vi "ECU Events Page.vi"(8 "error in (no error)":errorcluster, 11 "Node Ptr":T1 format="%.0x") -> (0 "error out":errorcluster)   [LabVIEW 2011, in "Engine Sim System Explorer.lvlib"]
uses:
  Engine Sim System Explorer.lvlib
  <vilib>/NI Veristand/Custom Device API/Custom Device Item Ref.ctl
  Shared/Engine Simulation Global.vi
  <vilib>/NI Veristand/Custom Device API/Get Item Property (Double).vi
  <vilib>/NI Veristand/Custom Device API/Set Item Property (Double).vi
  <vilib>/NI Veristand/Custom Device API/Custom Device API.lvlib
  Engine Simulation Shared.lvlib
panel:
  in  "FPGA Event Loop Rate (Hz)":dbl format="%#_p"
  in  "SHDocVw.IWebBrowser2":refnum<k7>(container)
  # "(Can be overriden per event on that event's page)"
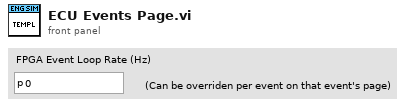
[diagram p1: front panel]
types:
  T1 = typedef "Custom Device API.lvlib/Custom Device Item Ref.ctl" = u64
  T2 = typedef "Custom Device API.lvlib/Custom Device Commands.ctl" = enum16{"Default", "Item renamed", "Shutdown", "Dynamic button pressed"}
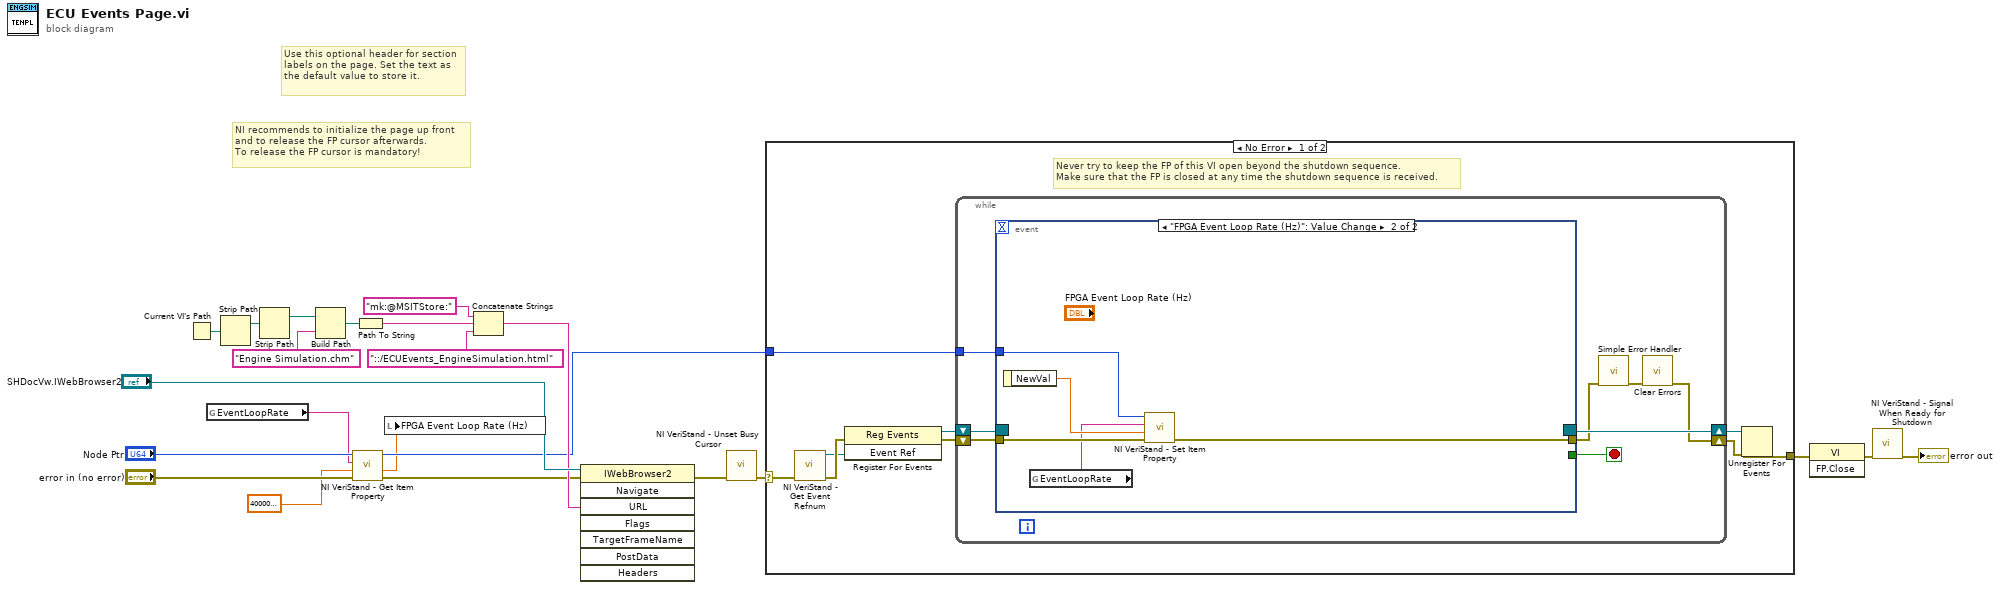
[diagram p0: block diagram]
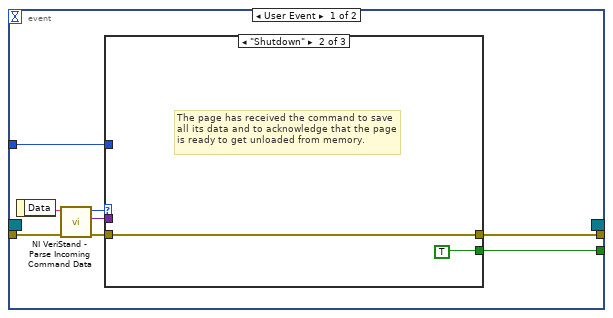
[diagram p2: hidden frame]
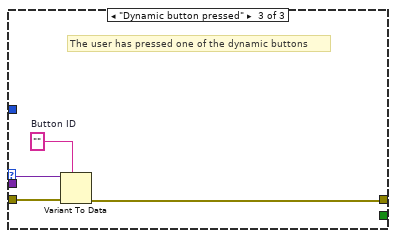
[diagram p4: hidden frame]
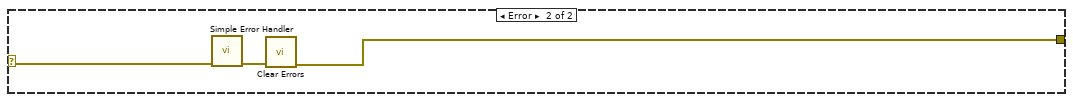
[diagram p5: hidden frame]
diagram:
  # "Use this optional header for section labels on the page. Set the text as the default value to store it."
  # "NI recommends to initialize the page up front\nand to release the FP cursor afterwards.\nTo release the FP cursor is mandatory!"
  n1 = Current VI's Path() -> (path=w9:path)
  n2 = global read "Engine Simulation Global.vi" "EventLoopRate"() -> (w3:string)
  n3 = Strip Path(path=w9) -> (stripped path=w10:path)  [unwired: 1 out]
  n4 = Strip Path(path=w10) -> (stripped path=w15:path)  [unwired: 1 out]
  n5 = Build Path(base path=w15, name or relative path="Engine Simulation.chm") -> (appended path=w13:path)
  n6 = call-poly <vilib>:"NI VeriStand - Get Item Property.vi"("error in (no error)"="error in (no error)", "Default Value"=40000000.0, "Property Name"=w3, "Item Ref in"="Node Ptr") -> ("error out"=w6:errorcluster, "Value"=w1:dbl, "Item Ref out"=w4:T1)  [unwired: 4 in, 1 out]
  n7 = Path To String(path=w13) -> (string=w12:string)
  n8 = local write "FPGA Event Loop Rate (Hz)"(w1) -> ()
  n9 = Concatenate Strings("mk:@MSITStore:" ("string"), w12, "::/ECUEvents_EngineSimulation.html" ("name or relative path")) -> (w7:string)
  n10 = invoke class="IWebBrowser2" method="Navigate"(reference="SHDocVw.IWebBrowser2", error in=w6, "URL"=w7) -> (error out=w19:errorcluster)  [unwired: 5 in, 7 out]
  n11 = call <vilib>:"NI VeriStand - Unset Busy Cursor.vi"("error in (no error)"=w19) -> ("error out"=w18:errorcluster)  [unwired: 10 out]
  n12 = case shown="No Error" w18 {
    selector: w18 -> [w23 w62]
    tunnel: [w28 w60] -> w22
    tunnel: w4 -> [w24 _]
    frame No Error {
      # "Never try to keep the FP of this VI open beyond the shutdown sequence.\nMake sure that the FP is closed at any time the shutdown sequence is received."
      n13 = call <vilib>:"NI VeriStand - Get Event Refnum.vi"("error in (no error)"=w23) -> ("error out"=w31:errorcluster, "Event Ref"=w27:refnum<user-event>)  [unwired: 9 out]
      n14 = register-events(error in=w31, w27) -> (reference out=w25:refnum<event-registration>, error out=w26:errorcluster)  [unwired: 1 in]
      n15 = while {
        tunnel: w24 -> [w35]
        shift-right: [w32] -> w29
        shift-left: w26 -> [w38]
        shift-right: [w39] -> w30
        shift-left: w25 -> [w37]
        stop <- w36 stop-if-true
        n16 = event shown="[1] \"FPGA Event Loop Rate (Hz)\": Value Change" {
          selector: w37 -> [_ _]
          dyn-events: [_ _] -> w39
          timeout: _ -> [_ _]
          tunnel: w38 -> [w47 w59]
          tunnel: [w43 _] -> w36
          tunnel: [w42 w55] -> w34
          tunnel: w35 -> [w41 w58]
          event User Event {
            n17 = event-data() -> ("Data"=w46:string)  [unwired: 1 out]
            n18 = call <vilib>:"NI VeriStand - Parse Incoming Command Data.vi"("error in (no error)"=w47, "Incoming data"=w46) -> ("error out"=w45:errorcluster, "Outgoing data"=w40:variant, "Action"=w44:T2)  [unwired: 7 out]
            n19 = case shown="\"Shutdown\"" w44 {
              tunnel: w45 -> [w48 w49 w54]
              tunnel: [_ TRUE _] -> w43
              tunnel: [w48 w49 w51] -> w42
              tunnel: w41 -> [_ _ _]
              tunnel: w40 -> [_ _ w53]
              frame "Default", Default {
              }
              frame "Shutdown" {
                # "The page has received the command to save all its data and to acknowledge that the page is ready to get unloaded from memory."
              }
              frame "Dynamic button pressed" {
                w52 = ""  # Button ID
                # "The user has pressed one of the dynamic buttons"
                n20 = Variant To Data(error in=w54, type=w52, Variant=w53) -> (error out=w51:errorcluster)  [unwired: 1 out]
              }
            }
          }
          event "FPGA Event Loop Rate (Hz)": Value Change {
            n21 = event-data() -> ("NewVal"=w57:dbl)  [unwired: 1 out]
            n22 = global read "Engine Simulation Global.vi" "EventLoopRate"() -> (w56:string)
            n23 = call-poly <vilib>:"NI VeriStand - Set Item Property.vi"("error in (no error)"=w59, "Value"=w57, "Property Name"=w56, "Item Ref in"=w58) -> ("error out"=w55:errorcluster)  [unwired: 5 in, 2 out]
          }
        }
        n24 = call <vilib>:"Simple Error Handler.vi"("error in (no error)"=w34) -> ("error out"=w33:errorcluster)  [unwired: 1 in, 7 out]
        n25 = call <vilib>:"Clear Errors.vi"("error in (no error)"=w33) -> ("error out"=w32:errorcluster)  [unwired: 6 out]
      }
      n26 = Unregister For Events(event registration refnum=w30, error in=w29) -> (error out=w28:errorcluster)
    }
    frame Error {
      n27 = call <vilib>:"Simple Error Handler.vi"("error in (no error)"=w62) -> ("error out"=w61:errorcluster)  [unwired: 1 in, 7 out]
      n28 = call <vilib>:"Clear Errors.vi"("error in (no error)"=w61) -> ("error out"=w60:errorcluster)  [unwired: 6 out]
    }
  }
  n29 = invoke class="VI" method="FP.Close"(error in=w22) -> (error out=w21:errorcluster)  [unwired: 2 in, 2 out]
  n30 = call <vilib>:"NI VeriStand - Signal When Ready for Shutdown.vi"("error in (no error)"=w21) -> ("error out"=→"error out":errorcluster)  [unwired: 10 out]
